vi "TSM Session Init and Cleanup.vi"(0 "TSM context":T1, 5 "Operation":T3, 7 "Power Line Frequency":T2=60.0 caption="Power Line Frequency (60Hz)" items=["50 Hertz"=50.0, "60 Hertz"=60.0]) -> (15 "error out":errorcluster)   [LabVIEW 2019]
uses:
  TSM Session Command.ctl
  <instrlib>/niDCPower/nidcpower.llb/niDCPower Power Line Frequency.ctl
  <vilib>/NI_TestStand_SemiconductorModule/NI_TestStand_Semiconductor_Module.lvlibp/PinMap/General/SemiconductorModuleContext.ctl
  <vilib>/NI_TestStand_SemiconductorModule/NI_TestStand_Semiconductor_Module.lvlibp
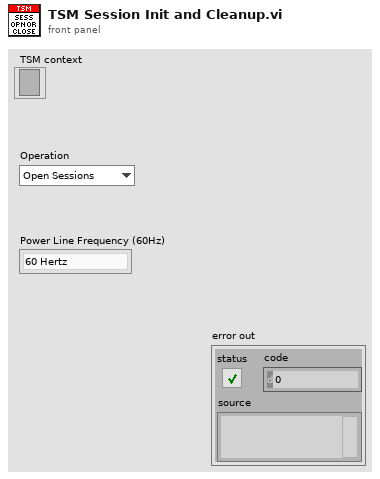
[diagram p1: front panel]
types:
  T1 = typedef "NI_TestStand_Semiconductor_Module.lvlibp/SemiconductorModuleContext.ctl" = refnum<k7>
  T2 = typedef "niDCPower Power Line Frequency.ctl" = dbl
  T3 = typedef "TSM Session Command.ctl" = enum16{"Open Sessions", "Close Sessions"}
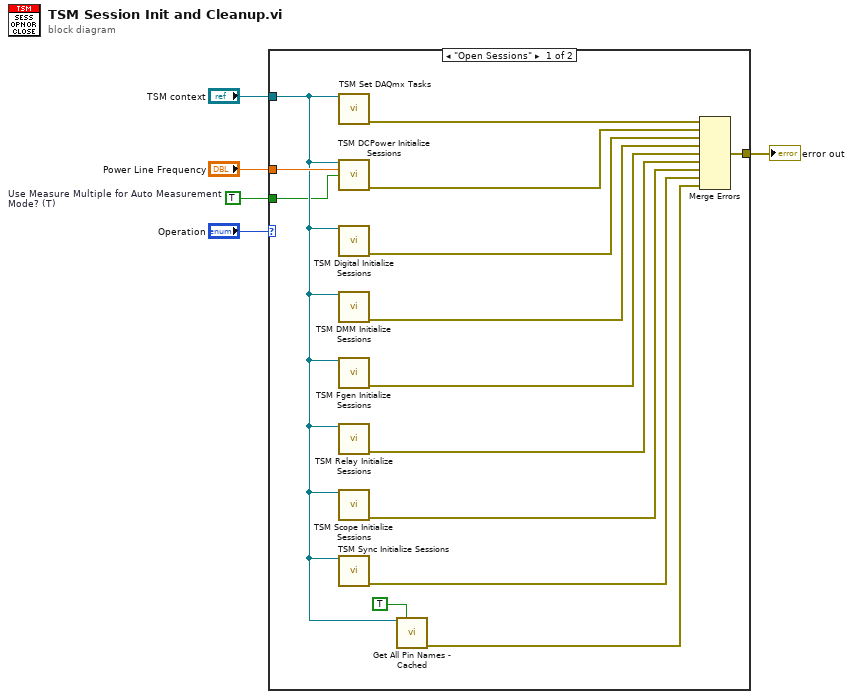
[diagram p0: block diagram]
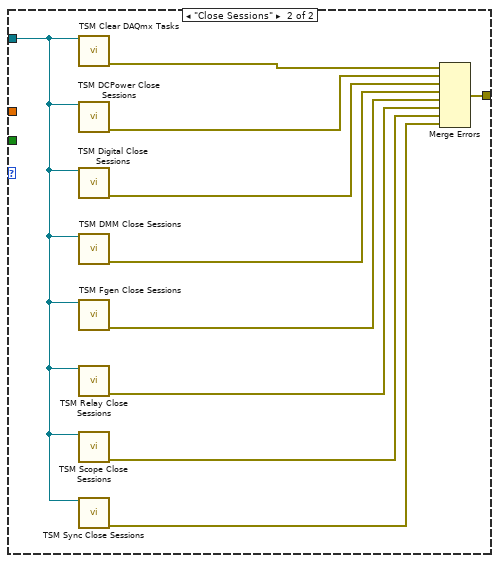
[diagram p2: hidden frame]
diagram:
  w1 = TRUE  # Use Measure Multiple for Auto Measurement Mode? (T)
  n1 = case shown="\"Open Sessions\"" "Operation" {
    tunnel: "TSM context" -> [w9 w20]
    tunnel: [w12 w29] -> w4
    tunnel: "Power Line Frequency" -> [w11 _]
    tunnel: w1 -> [w6 _]
    frame "Open Sessions" {
      n2 = call "TSM Set DAQmx Tasks.vi"("TSM context"=w9) -> ("error out"=w19:errorcluster)  [unwired: 14 in]
      n3 = call "TSM DCPower Initialize Sessions.vi"("TSM context"=w9, "Power Line Frequency"=w11, "Use Measure Multiple for Auto Measurement Mode? (T)"=w6) -> ("error out"=w18:errorcluster)  [unwired: 12 in]
      n4 = call "TSM Digital Initialize Sessions.vi"("TSM context"=w9) -> ("error out"=w17:errorcluster)  [unwired: 14 in]
      n5 = call "TSM DMM Initialize Sessions.vi"("TSM context"=w9) -> ("error out"=w16:errorcluster)  [unwired: 14 in]
      n6 = call "TSM Fgen Initialize Sessions.vi"("TSM context"=w9) -> ("error out"=w10:errorcluster)  [unwired: 14 in]
      n7 = call "TSM Relay Initialize Sessions.vi"("TSM context"=w9) -> ("error out"=w15:errorcluster)  [unwired: 14 in]
      n8 = call "TSM Scope Initialize Sessions.vi"("TSM context"=w9) -> ("error out"=w14:errorcluster)  [unwired: 14 in]
      n9 = call "TSM Sync Initialize Sessions.vi"("TSM context"=w9) -> ("error out"=w13:errorcluster)  [unwired: 14 in]
      n10 = call "Get All Pin Names - Cached.vi"("TSM Context in"=w9, "Reload Cache?"=TRUE) -> ("error out"=w8:errorcluster)  [unwired: 11 in, 2 out]
      n11 = Merge Errors(w19, w18, w17, w16, w10, w15, w14, w13, w8) -> (w12:errorcluster)
    }
    frame "Close Sessions" {
      n12 = call "TSM Clear DAQmx Tasks.vi"("TSM context"=w20) -> ("error out"=w28:errorcluster)  [unwired: 14 in]
      n13 = call "TSM DCPower Close Sessions.vi"("TSM context"=w20) -> ("error out"=w27:errorcluster)  [unwired: 14 in]
      n14 = call "TSM Digital Close Sessions.vi"("TSM context"=w20) -> ("error out"=w26:errorcluster)  [unwired: 14 in]
      n15 = call "TSM DMM Close Sessions.vi"("TSM context"=w20) -> ("error out"=w25:errorcluster)  [unwired: 14 in]
      n16 = call "TSM Fgen Close Sessions.vi"("TSM context"=w20) -> ("error out"=w21:errorcluster)  [unwired: 14 in]
      n17 = call "TSM Relay Close Sessions.vi"("TSM context"=w20) -> ("error out"=w24:errorcluster)  [unwired: 14 in]
      n18 = call "TSM Scope Close Sessions.vi"("TSM context"=w20) -> ("error out"=w23:errorcluster)  [unwired: 14 in]
      n19 = call "TSM Sync Close Sessions.vi"("TSM context"=w20) -> ("error out"=w22:errorcluster)  [unwired: 14 in]
      n20 = Merge Errors(w28, w27, w26, w25, w21, w24, w23, w22) -> (w29:errorcluster)
    }
  }
  "error out" <- w4
